vi "MsgUsuarioOK_CANCEL.vi"() -> ()   [LabVIEW 2018]
panel:
  in  "texto":string
  in  "OK":bool
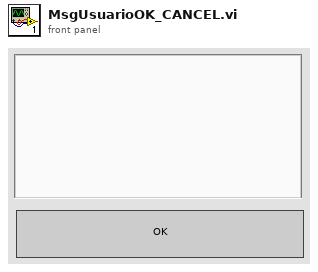
[diagram p1: front panel]
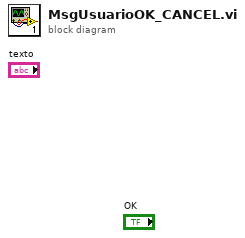
[diagram p0: block diagram]
diagram:
